vi "CThread Teleop Template.vi"() -> ()   [LabVIEW 2010]
uses:
  CLIB/CThread/XNodes/initializernode/CThread Initializer.xnode
  CLIB/CThread/Core/CThread Governor.vi
  Process All FTC Functions.vi
  Remote Interface/Remote Interface.lvlib
  FTC.lvlib
  CLIB/CThread/CThread.lvlib
panel:
  out "Enabled?":enum16{"Disabled", "Enabled"}(ring)
types:
  T1 = typedef "LVHSConnector.ctl" = cluster{"Hardware":string, "Flattened String":string}
  T2 = enum16{"Pressed", "Released", "Toggled", "Untoggled"}
  T3 = enum16{"None", "Left Button", "Right Button", "Enter Button"}
  T4 = enum16{"None", "Button 1", "Button 2", "Button 3", "Button 4", "Button 5", "Button 6", "Button 7", "Button 8", "Button 9", "Button 10", "Button 11", "Button 12", "POV Up", "POV Up Right", "POV Right", "POV Down Right", "POV Down", "POV Down Left", "POV Left", "POV Up Left"}
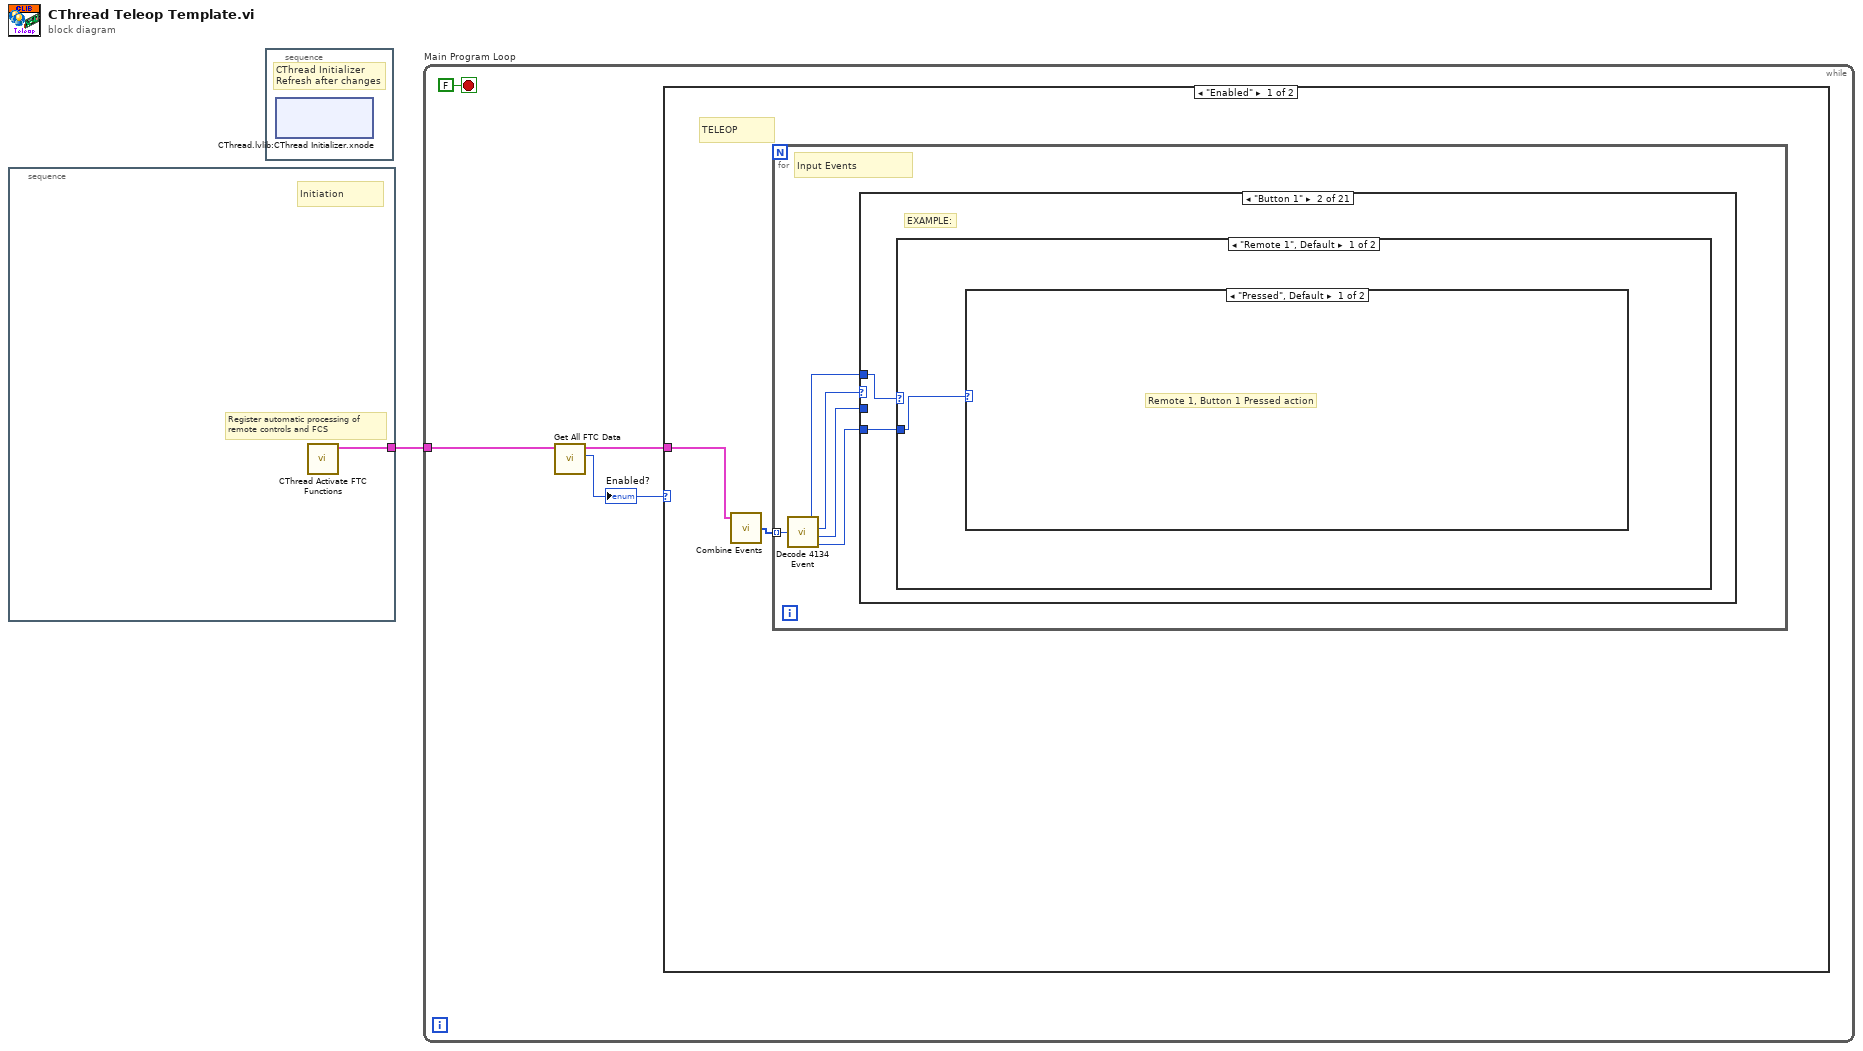
[diagram p0: block diagram]
diagram:
  n1 = stacked-sequence {
    tunnel: [w2] -> w1
    frame #0 {
      # "Register automatic processing of\nremote controls and FCS"
      # "Initiation"
      n2 = call "CThread Activate FTC Functions.vi"() -> ("NXT"=w2:T1)  [unwired: 11 in]
    }
  }
  n3 = stacked-sequence {
    frame #0 {
      # "CThread Initializer\nRefresh after changes"
      n4 = xnode "CThread.lvlib:CThread Initializer.xnode"() -> ()
    }
  }
  n5 = while "Main Program Loop" {
    tunnel: w1 -> [w18]
    stop <- FALSE stop-if-true
    n6 = call "Get All FTC Data.vi"("NXT"=w18) -> ("Enabled?"=w16:enum16{"Disabled", "Enabled"}, "NXT"=w17:T1)  [unwired: 3 in, 6 out]
    "Enabled?" <- w16
    n7 = case "disableCase" shown="\"Enabled\"" w16 {
      tunnel: w17 -> [w21 w35]
      frame "Enabled" {
        # "TELEOP"
        n8 = call "Combine Events.vi"("NXT"=w21) -> ("4134 Events"=w20:u8[])  [unwired: 3 in, 1 out]
        n9 = for {
          tunnel: w20 -> [w26] mode=indexing
          # "Input Events"
          n10 = call "Decode 4134 Event.vi"("4134 Event"=w26) -> ("4134 Event Type"=w23:T2, "NXT Button"=w24:T3, "FTC Button"=w25:T4, "Source"=w22:enum16{"NXT", "Remote 1", "Remote 2"})
          n11 = case shown="\"Button 1\"" w25 {
            tunnel: w24 -> [w28 _ _ _ _ _ _ _ _ _ _ _ _ _ _ _ _ _ _ _ _]
            tunnel: w23 -> [w27 w32 _ _ _ _ _ _ _ _ _ _ _ _ _ _ _ _ _ _ _]
            tunnel: w22 -> [w29 w33 _ _ _ _ _ _ _ _ _ _ _ _ _ _ _ _ _ _ _]
            frame "None", Default {
              n12 = case shown="\"NXT\"" w29 {
                tunnel: w28 -> [w31 _]
                tunnel: w27 -> [w30 _]
                frame "NXT" {
                  # "An NXT Button was pressed:"
                  n13 = case shown="\"None\", Default" w31 {
                    tunnel: w30 -> [_ _ _ _]
                    frame "None", Default {
                    }
                    frame "Left Button" {
                    }
                    frame "Right Button" {
                    }
                    frame "Enter Button" {
                    }
                  }
                }
                frame Default {
                  # "Invalid case, do nothing"
                }
              }
            }
            frame "Button 1" {
              # "EXAMPLE:"
              n14 = case shown="\"Remote 1\", Default" w33 {
                tunnel: w32 -> [w34 _]
                frame "Remote 1", Default {
                  n15 = case shown="\"Pressed\", Default" w34 {
                    frame "Pressed", Default {
                      # "Remote 1, Button 1 Pressed action"
                    }
                    frame "Released" {
                      # "Remote 1, Button 1 Released action"
                    }
                  }
                }
                frame "Remote 2" {
                }
              }
            }
            frame "Button 2" {
            }
            frame "Button 3" {
            }
            frame "Button 4" {
            }
            frame "Button 5" {
            }
            frame "Button 6" {
            }
            frame "Button 7" {
            }
            frame "Button 8" {
            }
            frame "Button 9" {
            }
            frame "Button 10" {
            }
            frame "Button 11" {
            }
            frame "Button 12" {
            }
            frame "POV Up" {
            }
            frame "POV Up Right" {
            }
            frame "POV Right" {
            }
            frame "POV Down Right" {
            }
            frame "POV Down" {
            }
            frame "POV Down Left" {
            }
            frame "POV Left" {
            }
            frame "POV Up Left" {
            }
          }
        }
      }
      frame "Disabled" {
        n16 = call <vilib>:"FTC Display Connection Status.vi"("NXT"=w35) -> ()  [unwired: 10 in, 1 out]
      }
    }
  }
